vi "log-channel-2-boolarray-and-names.vi"(6 "min_number_chan":i16=2, 8 "error in":errorcluster, 11 "Logging selection":T1) -> (0 "error out":errorcluster, 1 "Channel-Names":string[](array[string]), 2 "num_chan":i32, 3 "Log-Channel_select":bool[](array[boolean]))   [LabVIEW 2017]
uses:
  controls/logging_selection.ctl
  <vilib>/Utility/error.llb/DialogType.ctl
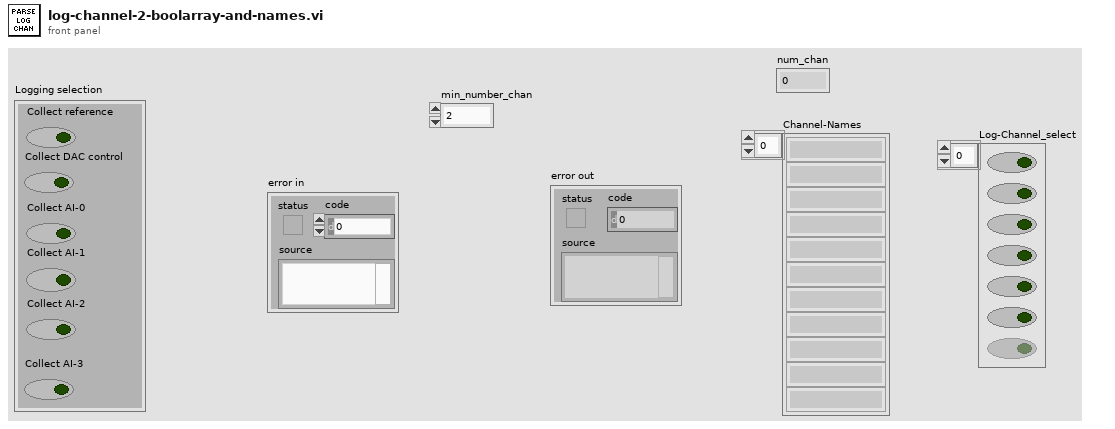
[diagram p1: front panel]
types:
  T1 = typedef "logging_selection.ctl" = cluster{"Collect reference":bool, "Collect DAC control":bool, "Collect AI-0":bool, "Collect AI-1":bool, "Collect AI-2":bool, "Collect AI-3":bool}
  T2 = typedef "DialogType.ctl" = u16
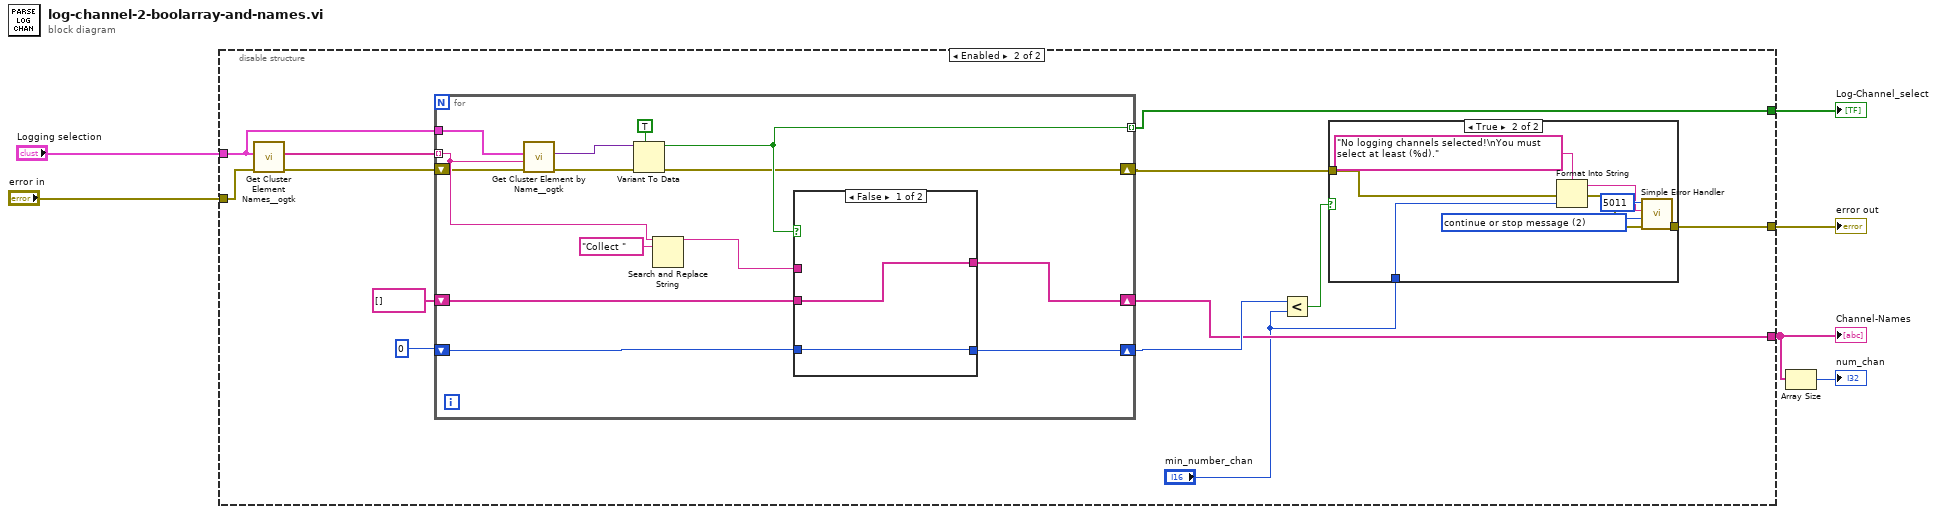
[diagram p0: block diagram]
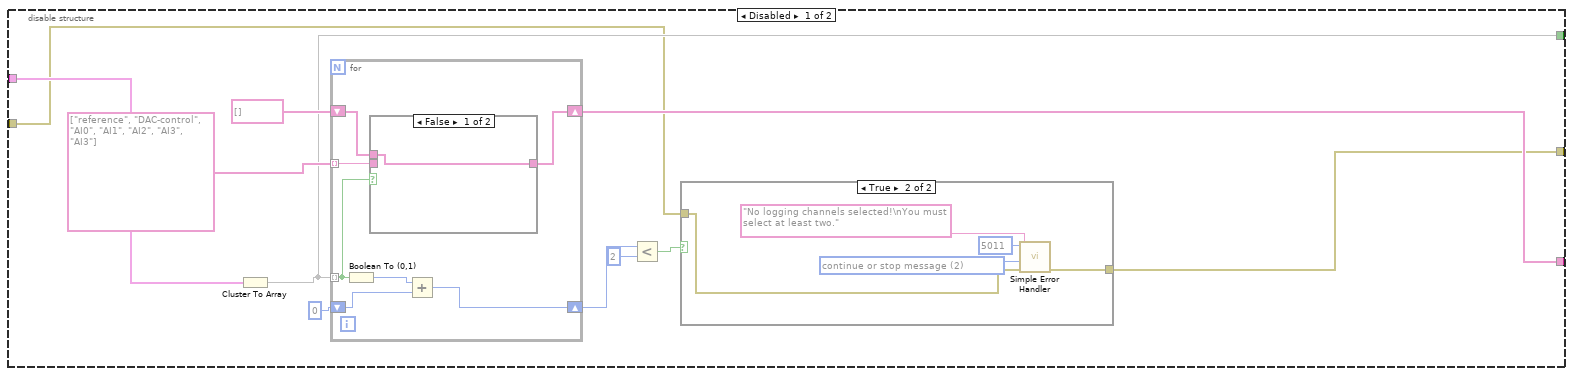
[diagram p2: hidden frame]
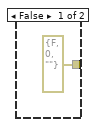
[diagram p3: hidden frame]
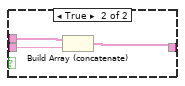
[diagram p4: hidden frame]
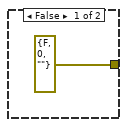
[diagram p5: hidden frame]
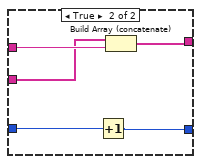
[diagram p6: hidden frame]
diagram:
  n1 = disable-structure shown="Enabled" {
    disable-tunnel: [w15 w37] -> w2
    disable-tunnel: "Logging selection" -> [w13 w41]
    disable-tunnel: [w12 w36] -> w5
    disable-tunnel: [w8 w38] -> w4
    disable-tunnel: "error in" -> [w7 w40]
    frame Disabled {
      n2 = Cluster To Array(cluster=w13) -> (array=w12:bool[])
      n3 = for {
        tunnel: w12 -> [w27] mode=indexing
        shift-right: [w29] -> w10
        shift-left: i16 0 -> [w28]
        tunnel: string[] ["reference", "DAC-control", "AI0", "AI1", "AI2", "AI3", "AI3"] -> [w26] mode=indexing
        shift-right: [w25] -> w15
        shift-left: string[] [] -> [w24]
        n4 = Boolean To (0,1)(Boolean=w27) -> (0, 1=w30:i16)
        n5 = case shown="False" w27 {
          tunnel: w26 -> [_ w34]
          tunnel: [w31 w33] -> w25
          tunnel: w24 -> [w31 w32]
          frame False {
          }
          frame True {
            n6 = Build Array (concatenate)(w32, w34) -> (w33:string[])
          }
        }
        n7 = Add(x=w30, y=w28) -> (x+y=w29:i16)
      }
      n8 = Less?(x=w10, y=i16 2) -> (x < y?=w11:bool)
      n9 = case shown="True" w11 {
        tunnel: [errorcluster {"status"=FALSE, "code"=0, "source"=""} ("error out") w21] -> w8
        tunnel: w7 -> [_ w20]
        frame False {
        }
        frame True {
          w23 = T2 2 items=["no dialog", "OK message", "continue or stop message", "OK message + warnings", "continue/stop + warnings"] ("type of dialog (OK msg:1)")
          n10 = call <vilib>:"Simple Error Handler.vi"("error code (no error:0)"=5011, "error source (\" \")"="No logging channels selected!\nYou must select at least two." ("error source (\" \")"), "type of dialog (OK msg:1)"=w23, "error in (no error)"=w20) -> ("error out"=w21:errorcluster)  [unwired: 1 in, 4 out]
        }
      }
    }
    frame Enabled {
      n11 = call <userlib>:"Get Cluster Element Names__ogtk.vi"("error in (no error)"=w40, "Cluster"=w41) -> ("error out"=w45:errorcluster, "Element Names"=w47:string[])  [unwired: 8 in]
      n12 = for {
        tunnel: w47 -> [w67] mode=indexing
        tunnel: w41 -> [w70]
        shift-right: [w64] -> w37
        shift-left: string[] [] -> [w63]
        tunnel: [w58] -> w36 mode=indexing
        shift-right: [w62] -> w39
        shift-left: i16 0 -> [w61]
        shift-right: [w57] -> w43
        shift-left: w45 -> [w60]
        n13 = call <userlib>:"Get Cluster Element by Name__ogtk.vi"("error in (no error)"=w60, "Element Name"=w67, "Cluster"=w70) -> ("error out"=w59:errorcluster, "VElement"=w69:variant)  [unwired: 6 in, 1 out]
        n14 = Variant To Data(error in=w59, type=TRUE, Variant=w69) -> (data=w58:bool, error out=w57:errorcluster)
        n15 = Search and Replace String(input string=w67, search string="Collect ") -> (result string=w65:string)  [unwired: 6 in, 3 out]
        n16 = case shown="False" w58 {
          tunnel: w65 -> [_ w77]
          tunnel: [w72 w76] -> w64
          tunnel: w63 -> [w72 w75]
          tunnel: w61 -> [w71 w74]
          tunnel: [w71 w73] -> w62
          frame False {
          }
          frame True {
            n17 = Increment(x=w74) -> (x+1=w73:i16)
            n18 = Build Array (concatenate)(w75, w77) -> (w76:string[])
          }
        }
      }
      n19 = Less?(x=w39, y="min_number_chan") -> (x < y?=w44:bool)
      n20 = case shown="True" w44 {
        tunnel: [errorcluster {"status"=FALSE, "code"=0, "source"=""} ("error out") w55] -> w38
        tunnel: w43 -> [_ w50]
        tunnel: "min_number_chan" -> [_ w51]
        frame False {
        }
        frame True {
          w56 = T2 2 items=["no dialog", "OK message", "continue or stop message", "OK message + warnings", "continue/stop + warnings"] ("type of dialog (OK msg:1)")
          n21 = Format Into String(format string="No logging channels selected!\nYou must select at least (%d)." ("error source (\" \")"), error in=w50, w51) -> (resulting string=w53:string, error out=w49:errorcluster)  [unwired: 1 in]
          n22 = call <vilib>:"Simple Error Handler.vi"("error code (no error:0)"=5011, "error source (\" \")"=w53, "type of dialog (OK msg:1)"=w56, "error in (no error)"=w49) -> ("error out"=w55:errorcluster)  [unwired: 1 in, 4 out]
        }
      }
    }
  }
  "Channel-Names" <- w2
  "Log-Channel_select" <- w5
  "error out" <- w4
  n23 = Array Size(array=w2) -> (size(s)=→"num_chan":i32)
